vi "Autonomous Independent.vi"   [LabVIEW 2013]
doc: "This VI is called when autonomous begins, and will automatically be terminated when autonomous ends. You can carry out timed or sensor driven robot movement independently without needing to return to the caller."
uses:
  <vilib>/Rock Robotics/WPI/Relay/WPI_RelayValue.ctl
  <vilib>/Rock Robotics/WPI/Solenoid/WPI_SolenoidValue.ctl
  Robot Global Data.vi
  <vilib>/Rock Robotics/WPI/RobotDrive/WPI_RobotDriveGetSetRefNum.vi
  <vilib>/Rock Robotics/WPI/RobotDrive/WPI_RobotDriveArcadeDrive_Standard(NoSaturation).vi
  <vilib>/Rock Robotics/WPI/Solenoid/WPI_SolenoidSetEnum.vi
  <vilib>/Rock Robotics/WPI/Joystick/WPI_JoystickGetSetRefNum.vi
panel:
  # "Be sure to right-click and choose Data Operations>>Make Current Value default if you want to save the array values with the VI"
types:
  T1 = typedef "WPI_JoystickDevRef.ctl" = cluster{"Device":T2}
  T2 = typedef "WPI_JoystickDeviceEnum.ctl" = enum16{"USB 1", "USB 2", "USB 3", "USB 4", "Kinect 1", "Kinect 2"}
  T3 = cluster{"axis 1 (x)":dbl, "axis 2 (y)":dbl, "axis 3 (throttle)":dbl, "axis 4":dbl, "axis 5":dbl, "axis 6":dbl}
  T4 = typedef "WPI_RobotDriveDevRef.ctl" = cluster{"DevStatus":errorcluster, "Motors[]":T5[], "Square Inputs":bool, "Max Output":dbl, "Isochronous":bool}
  T5 = typedef "WPI_MotorControlDeviceRef.ctl" = cluster{"DeviceStatus":errorcluster, "Type":enum16{"PWM", "CAN"}, "PWM":cluster{"Digital Module":T6, "PWM Channel":T7, "DeadBand":T8}, "CAN":cluster{"Device Number":u8, "Control Mode":T9, "Semaphore":T10, "Max Vout":dbl}, "Invert":bool, "TransformRef":T11, "InvTransformRef":T11}
  T6 = typedef "FPGA_TypedefDigitalModule.ctl" = enum16{"Digital Module 1", "Digital Module 2"}
  T7 = typedef "FPGA_DIOPWMChannel.ctl" = enum8{"PWM 1", "PWM 2", "PWM 3", "PWM 4", "PWM 5", "PWM 6", "PWM 7", "PWM 8", "PWM 9", "PWM 10", "Invalid"}
  T8 = typedef "WPI_PWMDeadband.ctl" = cluster{"Name":string, "maxPositivePwm":i32, "minPositivePwm":i32, "centerPwm":i32, "maxNegativePwm":i32, "minNegativePwm":i32, "angularRange":u16}
  T9 = typedef "WPI_CANJaguar_ControlMode.ctl" = enum8{"Percent VBus", "Current", "Speed", "Position", "Voltage"}
  T10 = typedef "Semaphore RefNum" = refnum<k1>
  T11 = typedef "WPI_PWMTransform_ConPane.ctl" = refnum<vi>
  T12 = typedef "WPI_RelayDevRef.ctl" = cluster{"DevStatus":errorcluster, "Relay Channel":T13, "Digital Module":T6, "Relay Direction":T14}
  T13 = typedef "FPGA_DIORelayChannel.ctl" = enum8{"Relay 1", "Relay 2", "Relay 3", "Relay 4", "Relay 5", "Relay 6", "Relay 7", "Relay 8", "Invalid"}
  T14 = typedef "WPI_RelayDirection.ctl" = enum16{"Both directions", "Forward only", "Reverse only"}
  T15 = typedef "WPI_SolenoidDevRef.ctl" = cluster{"DevStatus":errorcluster, "Solenoid Module":T16, "Forward Solenoid Channel":T17, "Reverse Solenoid Channel":T17}
  T16 = typedef "FPGA_TypedefSolenoidModule.ctl" = enum16{"Solenoid Module 1", "Solenoid Module 2"}
  T17 = typedef "WPI_SolenoidChannel.ctl" = enum8{"Solenoid 1", "Solenoid 2", "Solenoid 3", "Solenoid 4", "Solenoid 5", "Solenoid 6", "Solenoid 7", "Solenoid 8", "Invalid"}
  T18 = typedef "WPI_SolenoidValue.ctl" = enum16{"Off", "On", "Forward", "Reverse"}
  T19 = typedef "WPI_RelayValue.ctl" = enum16{"Off", "On", "Forward", "Reverse"}
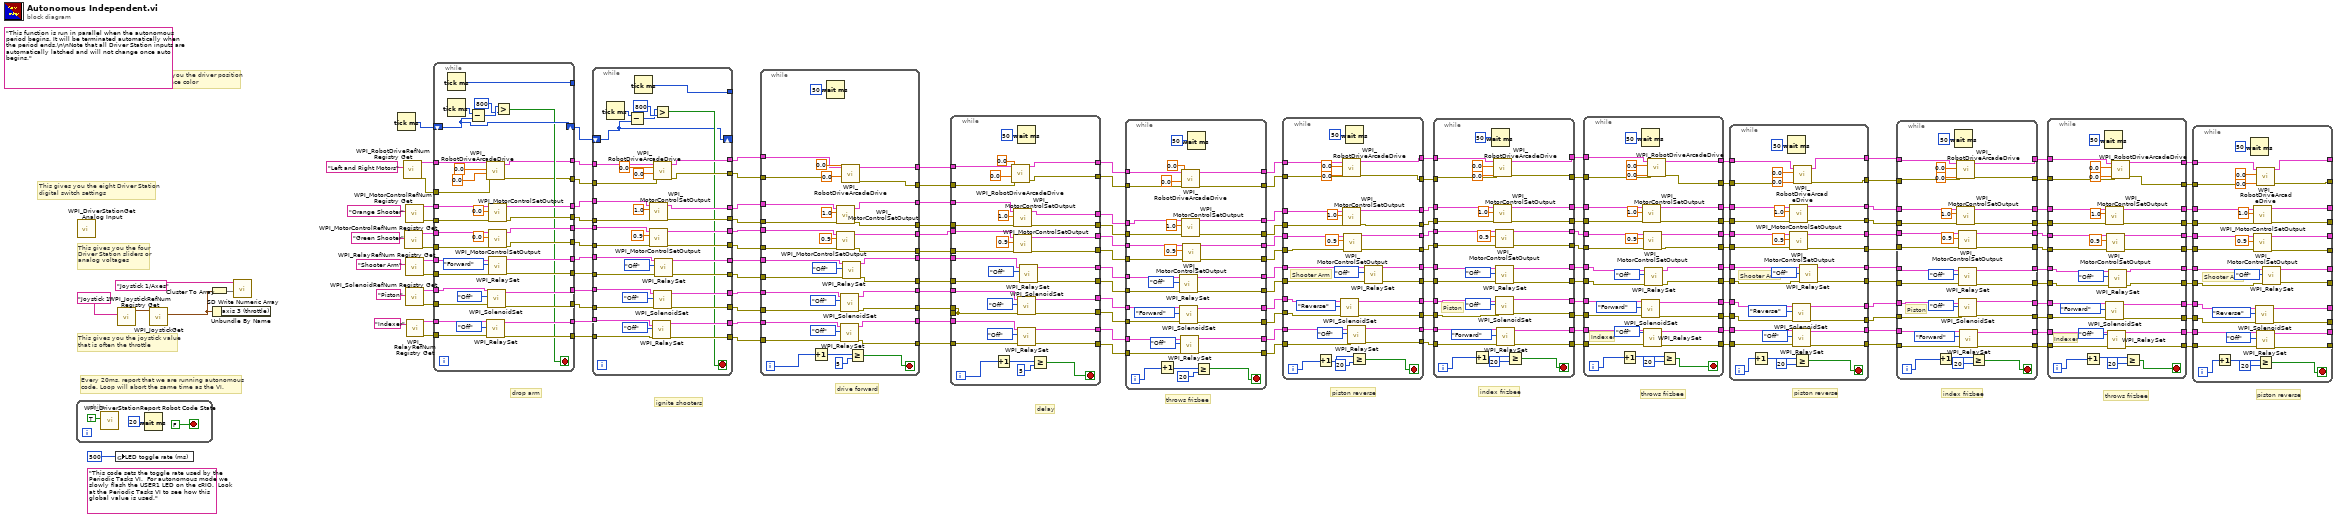
[diagram p0: block diagram]
diagram:
  (unwired) "This code sets the toggle rate used by the Periodic Tasks VI.  For autonomous mode we slowly flash the USER1 LED on the cRIO.  Look at the Periodic Tasks VI to see how this global value is used."
  (unwired) "This function is run in parallel when the autonomous period begins. It will be terminated automatically when the period ends.\n\nNote that all Driver Station inputs are automatically latched and will not change once auto begins."
  # "piston reverse"
  # "throws frizbee"
  # "index frizbee"
  # "drive forward"
  # "delay"
  # "ignite shooters"
  # "drop arm"
  # "piston reverse"
  # "throws frizbee"
  # "index frizbee"
  # "piston reverse"
  # "throws frizbee"
  # "This tells you the driver position\nand alliance color"
  # "Every 20ms, report that we are running autonomous\ncode. Loop will abort the same time as the VI."
  # "This gives you the joystick value\nthat is often the throttle"
  # "This gives you the eight Driver Station\ndigital switch settings"
  # "This gives you the four\nDriver Station sliders or\nanalog voltages"
  n1 = while {
    stop <- FALSE stop-if-true
    n2 = call <vilib>:"WPI_DriverStationReport Robot Code State.vi"("Autonomous"=TRUE) -> ()  [unwired: 10 in, 1 out]
    n3 = Wait (ms)(milliseconds to wait=u32 20) -> ()  [unwired: 1 out]
  }
  n4 = call <vilib>:"WPI_DriverStationGet Analog Input.vi"() -> ()  [unwired: 12 out]
  n5 = global write "Robot Global Data.vi" "LED toggle rate (ms)"(u32 500 ("LED ms toggle rate")) -> ()
  n6 = call <vilib>:"WPI_JoystickRefNum Registry Get.vi"("refnum name"="Joystick 1") -> ("JoystickDevRef"=w157:T1)  [unwired: 1 in, 9 out]
  n7 = call <vilib>:"WPI_JoystickGet.vi"("JoystickDevRef"=w157) -> ("Axes"=w154:T3)  [unwired: 1 in, 5 out]
  n8 = Cluster To Array(cluster=w154) -> (array=w155:dbl[])
  n9 = Unbundle By Name(w154) -> ()  [unwired: 1 out]
  n10 = call <vilib>:"SD Write Numeric Array.vi"("Numeric Array"=w155, "Name"="Joystick 1/Axes") -> ()  [unwired: 8 in, 2 out]
  n11 = Tick Count (ms)() -> (millisecond timer value=w148:u32)
  n12 = call <vilib>:"WPI_RobotDriveRefNum Registry Get.vi"("refnum name"="Left and Right Motors") -> ("error out"=w152:errorcluster, "RobotDriveDevRef"=w151:T4)  [unwired: 9 in]
  n13 = call <vilib>:"WPI_MotorControlRefNum Registry Get.vi"("refnum name"="Green Shooter") -> ("error out"=w138:errorcluster, "MotorControlDevRef"=w141:T5)  [unwired: 9 in]
  n14 = call <vilib>:"WPI_MotorControlRefNum Registry Get.vi"("refnum name"="Orange Shooter") -> ("error out"=w137:errorcluster, "MotorControlDevRef"=w140:T5)  [unwired: 9 in]
  n15 = call <vilib>:"WPI_RelayRefNum Registry Get.vi"("refnum name"="Shooter Arm") -> ("error out"=w139:errorcluster, "RelayDevRef"=w142:T12)  [unwired: 9 in]
  n16 = call <vilib>:"WPI_SolenoidRefNum Registry Get.vi"("refnum name"="Piston") -> ("error out"=w144:errorcluster, "SolenoidDevRef"=w143:T15)  [unwired: 9 in]
  n17 = call <vilib>:"WPI_RelayRefNum Registry Get.vi"("refnum name"="Indexer") -> ("error out"=w147:errorcluster, "RelayDevRef"=w146:T12)  [unwired: 9 in]
  n18 = while {
    tunnel: w137 -> [w198]
    tunnel: w138 -> [w197]
    tunnel: w139 -> [w196]
    tunnel: w140 -> [w188]
    tunnel: w141 -> [w185]
    tunnel: w142 -> [w195]
    tunnel: [w193] -> w129
    tunnel: [w192] -> w130
    tunnel: [w191] -> w128
    tunnel: [w190] -> w127
    tunnel: [w189] -> w126
    tunnel: w143 -> [w169]
    tunnel: w144 -> [w183]
    tunnel: [w182] -> w125
    tunnel: [w181] -> w124
    tunnel: w146 -> [w180]
    tunnel: [w178] -> w123
    tunnel: [w177] -> w122
    tunnel: w147 -> [w179]
    tunnel: [w187] -> w131
    shift-right: [w175] -> w61
    shift-left: w148 -> [w175]
    tunnel: [w171] -> _
    tunnel: w151 -> [w167]
    tunnel: [w166] -> w133
    tunnel: [w163] -> w132
    tunnel: w152 -> [w162]
    stop <- w172 stop-if-true
    n19 = Tick Count (ms)() -> (millisecond timer value=w170:u32)
    n20 = Tick Count (ms)() -> (millisecond timer value=w171:u32)
    n21 = Subtract(x=w170, y=w175) -> (x-y=w174:u32)
    n22 = call-poly <vilib>:"WPI_RobotDriveArcadeDrive.vi"("error in (no error)"=w162, "Y axis value"=0.0 ("X axis value"), "X axis value"=0.0, "RobotDriveDevRef"=w167) -> ("error out"=w163:errorcluster, "RobotDriveDevRef"=w166:T4)  [unwired: 5 in, 1 out]
    n23 = call <vilib>:"WPI_RelaySet.vi"("error in (no error)"=w179, "RelayValue"=WPI_RelayValue."Off", "RelayDevRef"=w180) -> ("error out"=w177:errorcluster, "RelayDevRef"=w178:T12)  [unwired: 7 in]
    n24 = call-poly <vilib>:"WPI_SolenoidSet.vi"("error in (no error)"=w183, "Value"=WPI_SolenoidValue."Off", "SolenoidDevRef"=w169) -> ("error out"=w181:errorcluster, "SolenoidDevRef"=w182:T15)  [unwired: 7 in]
    n25 = call <vilib>:"WPI_MotorControlSetOutput.vi"("error in (no error)"=w198, "Output"=0.0, "MotorControlDevRef"=w188) -> ("error out"=w192:errorcluster, "MotorControlDevRef"=w187:T5)  [unwired: 6 in, 1 out]
    n26 = call <vilib>:"WPI_MotorControlSetOutput.vi"("error in (no error)"=w197, "Output"=0.0, "MotorControlDevRef"=w185) -> ("error out"=w191:errorcluster, "MotorControlDevRef"=w193:T5)  [unwired: 6 in, 1 out]
    n27 = call <vilib>:"WPI_RelaySet.vi"("error in (no error)"=w196, "RelayValue"=WPI_RelayValue."Forward", "RelayDevRef"=w195) -> ("error out"=w189:errorcluster, "RelayDevRef"=w190:T12)  [unwired: 7 in]
    n28 = Greater?(x=w174, y=u32 800) -> (0:w172:bool)
  }
  n29 = while {
    tunnel: w131 -> [w233]
    tunnel: w130 -> [w232]
    tunnel: w129 -> [w231]
    tunnel: w128 -> [w230]
    tunnel: [w229] -> w42
    tunnel: [w228] -> w41
    tunnel: [w227] -> w39
    tunnel: [w226] -> w40
    tunnel: w127 -> [w222]
    tunnel: w126 -> [w221]
    tunnel: [w220] -> w51
    tunnel: [w219] -> w52
    tunnel: w125 -> [w218]
    tunnel: w124 -> [w217]
    tunnel: w123 -> [w216]
    tunnel: w122 -> [w215]
    tunnel: [w214] -> w60
    tunnel: [w213] -> w59
    tunnel: [w212] -> w56
    tunnel: [w211] -> w55
    tunnel: w133 -> [w210]
    tunnel: [w209] -> w44
    tunnel: w132 -> [w206]
    tunnel: [w205] -> w43
    tunnel: [w204] -> _
    shift-right: [w199] -> _
    shift-left: w61 -> [w199]
    stop <- w200 stop-if-true
    n30 = Tick Count (ms)() -> (millisecond timer value=w203:u32)
    n31 = Subtract(x=w203, y=w199) -> (x-y=w201:u32)
    n32 = Tick Count (ms)() -> (millisecond timer value=w204:u32)
    n33 = call <vilib>:"WPI_MotorControlSetOutput.vi"("error in (no error)"=w232, "Output"=1.0, "MotorControlDevRef"=w233) -> ("error out"=w228:errorcluster, "MotorControlDevRef"=w229:T5)  [unwired: 6 in, 1 out]
    n34 = call <vilib>:"WPI_MotorControlSetOutput.vi"("error in (no error)"=w230, "Output"=0.9, "MotorControlDevRef"=w231) -> ("error out"=w227:errorcluster, "MotorControlDevRef"=w226:T5)  [unwired: 6 in, 1 out]
    n35 = call <vilib>:"WPI_RelaySet.vi"("error in (no error)"=w215, "RelayValue"=WPI_RelayValue."Off", "RelayDevRef"=w216) -> ("error out"=w213:errorcluster, "RelayDevRef"=w214:T12)  [unwired: 7 in]
    n36 = call-poly <vilib>:"WPI_SolenoidSet.vi"("error in (no error)"=w217, "Value"=WPI_SolenoidValue."Off", "SolenoidDevRef"=w218) -> ("error out"=w212:errorcluster, "SolenoidDevRef"=w211:T15)  [unwired: 7 in]
    n37 = Greater?(x=w201, y=u32 800) -> (0:w200:bool)
    n38 = call-poly <vilib>:"WPI_RobotDriveArcadeDrive.vi"("error in (no error)"=w206, "Y axis value"=0.0, "X axis value"=0.0, "RobotDriveDevRef"=w210) -> ("error out"=w205:errorcluster, "RobotDriveDevRef"=w209:T4)  [unwired: 5 in, 1 out]
    n39 = call <vilib>:"WPI_RelaySet.vi"("error in (no error)"=w221, "RelayValue"=WPI_RelayValue."Off", "RelayDevRef"=w222) -> ("error out"=w219:errorcluster, "RelayDevRef"=w220:T12)  [unwired: 7 in]
  }
  n40 = while {
    tunnel: w60 -> [w264]
    tunnel: w59 -> [w263]
    tunnel: [w262] -> w58
    tunnel: [w261] -> w57
    tunnel: w56 -> [w260]
    tunnel: w55 -> [w259]
    tunnel: [w258] -> w54
    tunnel: [w257] -> w53
    tunnel: w52 -> [w256]
    tunnel: w51 -> [w255]
    tunnel: [w254] -> w50
    tunnel: [w253] -> w49
    tunnel: [w252] -> w48
    tunnel: [w251] -> w47
    tunnel: [w250] -> w46
    tunnel: [w249] -> w45
    tunnel: w44 -> [w247]
    tunnel: w43 -> [w246]
    tunnel: w42 -> [w245]
    tunnel: w41 -> [w244]
    tunnel: w40 -> [w243]
    tunnel: w39 -> [w242]
    tunnel: [w241] -> w38
    tunnel: [w240] -> w37
    i -> [w237]
    stop <- w236 stop-if-true
    n41 = Increment(x=w237) -> (x+1=w238:i32)
    n42 = Wait (ms)(milliseconds to wait=u32 50) -> ()  [unwired: 1 out]
    n43 = call <vilib>:"WPI_MotorControlSetOutput.vi"("error in (no error)"=w244, "Output"=1.0, "MotorControlDevRef"=w245) -> ("error out"=w249:errorcluster, "MotorControlDevRef"=w250:T5)  [unwired: 6 in, 1 out]
    n44 = call <vilib>:"WPI_MotorControlSetOutput.vi"("error in (no error)"=w242, "Output"=0.9, "MotorControlDevRef"=w243) -> ("error out"=w252:errorcluster, "MotorControlDevRef"=w251:T5)  [unwired: 6 in, 1 out]
    n45 = call <vilib>:"WPI_RelaySet.vi"("error in (no error)"=w263, "RelayValue"=WPI_RelayValue."Off", "RelayDevRef"=w264) -> ("error out"=w261:errorcluster, "RelayDevRef"=w262:T12)  [unwired: 7 in]
    n46 = call-poly <vilib>:"WPI_SolenoidSet.vi"("error in (no error)"=w260, "Value"=WPI_SolenoidValue."Off", "SolenoidDevRef"=w259) -> ("error out"=w257:errorcluster, "SolenoidDevRef"=w258:T15)  [unwired: 7 in]
    n47 = call-poly <vilib>:"WPI_RobotDriveArcadeDrive.vi"("error in (no error)"=w246, "Y axis value"=0.0, "X axis value"=0.0, "RobotDriveDevRef"=w247) -> ("error out"=w240:errorcluster, "RobotDriveDevRef"=w241:T4)  [unwired: 5 in, 1 out]
    n48 = call <vilib>:"WPI_RelaySet.vi"("error in (no error)"=w256, "RelayValue"=WPI_RelayValue."Off", "RelayDevRef"=w255) -> ("error out"=w253:errorcluster, "RelayDevRef"=w254:T12)  [unwired: 7 in]
    n49 = Greater Or Equal?(x=w238, y=5) -> (x >= y?=w236:bool)
  }
  n50 = while {
    tunnel: [w288] -> w102
    tunnel: [w289] -> w103
    tunnel: [w290] -> w104
    tunnel: [w291] -> w105
    tunnel: [w292] -> w106
    tunnel: [w293] -> w107
    tunnel: [w294] -> w108
    tunnel: [w295] -> w109
    tunnel: [w296] -> w110
    tunnel: [w297] -> w111
    tunnel: [w285] -> w112
    tunnel: [w284] -> w113
    tunnel: w38 -> [w283]
    tunnel: w37 -> [w282]
    tunnel: w45 -> [w281]
    tunnel: w46 -> [w280]
    tunnel: w48 -> [w279]
    tunnel: w47 -> [w278]
    tunnel: w49 -> [w277]
    tunnel: w50 -> [w276]
    tunnel: w54 -> [w275]
    tunnel: [w272] -> _
    tunnel: w58 -> [w274]
    tunnel: w57 -> [w273]
    tunnel: w53 -> [w272]
    i -> [w304]
    stop <- w303 stop-if-true
    n51 = Increment(x=w304) -> (x+1=w306:i32)
    n52 = call-poly <vilib>:"WPI_RobotDriveArcadeDrive.vi"("error in (no error)"=w282, "Y axis value"=0.0, "X axis value"=0.0, "RobotDriveDevRef"=w283) -> ("error out"=w284:errorcluster, "RobotDriveDevRef"=w285:T4)  [unwired: 5 in, 1 out]
    n53 = call <vilib>:"WPI_MotorControlSetOutput.vi"("error in (no error)"=w281, "Output"=1.0, "MotorControlDevRef"=w280) -> ("error out"=w289:errorcluster, "MotorControlDevRef"=w288:T5)  [unwired: 6 in, 1 out]
    n54 = call <vilib>:"WPI_MotorControlSetOutput.vi"("error in (no error)"=w279, "Output"=0.9, "MotorControlDevRef"=w278) -> ("error out"=w291:errorcluster, "MotorControlDevRef"=w290:T5)  [unwired: 6 in, 1 out]
    n55 = Wait (ms)(milliseconds to wait=u32 50) -> ()  [unwired: 1 out]
    n56 = call <vilib>:"WPI_RelaySet.vi"("error in (no error)"=w273, "RelayValue"=WPI_RelayValue."Off", "RelayDevRef"=w274) -> ("error out"=w297:errorcluster, "RelayDevRef"=w296:T12)  [unwired: 7 in]
    n57 = call-poly <vilib>:"WPI_SolenoidSet.vi"("error in (no error)"=w272, "Value"=WPI_SolenoidValue."Off", "SolenoidDevRef"=w275) -> ("error out"=w295:errorcluster, "SolenoidDevRef"=w294:T15)  [unwired: 7 in]
    n58 = call <vilib>:"WPI_RelaySet.vi"("error in (no error)"=w277, "RelayValue"=WPI_RelayValue."Off", "RelayDevRef"=w276) -> ("error out"=w293:errorcluster, "RelayDevRef"=w292:T12)  [unwired: 7 in]
    n59 = Greater Or Equal?(x=w306, y=5) -> (x >= y?=w303:bool)
  }
  n60 = while {
    tunnel: w104 -> [w328]
    tunnel: w103 -> [w343]
    tunnel: w105 -> [w342]
    tunnel: w106 -> [w326]
    tunnel: [w324] -> w62
    tunnel: w107 -> [w325]
    tunnel: [w323] -> w70
    tunnel: [w341] -> w68
    tunnel: [w340] -> w69
    tunnel: [w339] -> w66
    tunnel: [w338] -> w67
    tunnel: w108 -> [w315]
    tunnel: w109 -> [w337]
    tunnel: [w336] -> w64
    tunnel: [w335] -> w65
    tunnel: [w319] -> w78
    tunnel: w110 -> [w321]
    tunnel: w111 -> [w320]
    tunnel: [w318] -> w79
    tunnel: w102 -> [w330]
    tunnel: w112 -> [w313]
    tunnel: w113 -> [w312]
    tunnel: [w311] -> w114
    tunnel: [w310] -> w115
    i -> [w334]
    stop <- w331 stop-if-true
    n61 = Increment(x=w334) -> (x+1=w333:i32)
    n62 = call <vilib>:"WPI_RelaySet.vi"("error in (no error)"=w325, "RelayValue"=WPI_RelayValue."Off", "RelayDevRef"=w326) -> ("error out"=w323:errorcluster, "RelayDevRef"=w324:T12)  [unwired: 7 in]
    n63 = call-poly <vilib>:"WPI_SolenoidSet.vi"("error in (no error)"=w337, "Value"=WPI_SolenoidValue."Forward", "SolenoidDevRef"=w315) -> ("error out"=w335:errorcluster, "SolenoidDevRef"=w336:T15)  [unwired: 7 in]
    n64 = call <vilib>:"WPI_RelaySet.vi"("error in (no error)"=w320, "RelayValue"=WPI_RelayValue."Off", "RelayDevRef"=w321) -> ("error out"=w318:errorcluster, "RelayDevRef"=w319:T12)  [unwired: 7 in]
    n65 = call-poly <vilib>:"WPI_RobotDriveArcadeDrive.vi"("error in (no error)"=w312, "Y axis value"=0.0, "X axis value"=0.0, "RobotDriveDevRef"=w313) -> ("error out"=w310:errorcluster, "RobotDriveDevRef"=w311:T4)  [unwired: 5 in, 1 out]
    n66 = call <vilib>:"WPI_MotorControlSetOutput.vi"("error in (no error)"=w343, "Output"=1.0, "MotorControlDevRef"=w330) -> ("error out"=w338:errorcluster, "MotorControlDevRef"=w339:T5)  [unwired: 6 in, 1 out]
    n67 = call <vilib>:"WPI_MotorControlSetOutput.vi"("error in (no error)"=w342, "Output"=0.9, "MotorControlDevRef"=w328) -> ("error out"=w340:errorcluster, "MotorControlDevRef"=w341:T5)  [unwired: 6 in, 1 out]
    n68 = Wait (ms)(milliseconds to wait=u32 50) -> ()  [unwired: 1 out]
    n69 = Greater Or Equal?(x=w333, y=20) -> (x >= y?=w331:bool)
  }
  n70 = while {
    tunnel: w62 -> [w357]
    tunnel: [w355] -> w63
    tunnel: w64 -> [w352]
    tunnel: w65 -> [w376]
    tunnel: w66 -> [w366]
    tunnel: w67 -> [w365]
    tunnel: w68 -> [w364]
    tunnel: w69 -> [w378]
    tunnel: w70 -> [w356]
    tunnel: [w354] -> w75
    tunnel: [w377] -> w76
    tunnel: [w375] -> w77
    tunnel: [w374] -> w71
    tunnel: [w373] -> w74
    tunnel: [w372] -> w72
    tunnel: [w371] -> w73
    tunnel: [w359] -> w80
    tunnel: w78 -> [w361]
    tunnel: [w358] -> w81
    tunnel: w79 -> [w360]
    tunnel: w114 -> [w350]
    tunnel: w115 -> [w349]
    tunnel: [w346] -> w116
    tunnel: [w345] -> w117
    i -> [w370]
    stop <- w368 stop-if-true
    # "Shooter Arm"
    n71 = Increment(x=w370) -> (x+1=w369:i32)
    n72 = call-poly <vilib>:"WPI_SolenoidSet.vi"("error in (no error)"=w376, "Value"=WPI_SolenoidValue."Reverse", "SolenoidDevRef"=w352) -> ("error out"=w375:errorcluster, "SolenoidDevRef"=w377:T15)  [unwired: 7 in]
    n73 = call-poly <vilib>:"WPI_RobotDriveArcadeDrive.vi"("error in (no error)"=w349, "Y axis value"=0.0, "X axis value"=0.0, "RobotDriveDevRef"=w350) -> ("error out"=w345:errorcluster, "RobotDriveDevRef"=w346:T4)  [unwired: 5 in, 1 out]
    n74 = call <vilib>:"WPI_MotorControlSetOutput.vi"("error in (no error)"=w365, "Output"=1.0, "MotorControlDevRef"=w366) -> ("error out"=w373:errorcluster, "MotorControlDevRef"=w374:T5)  [unwired: 6 in, 1 out]
    n75 = call <vilib>:"WPI_MotorControlSetOutput.vi"("error in (no error)"=w378, "Output"=0.9, "MotorControlDevRef"=w364) -> ("error out"=w371:errorcluster, "MotorControlDevRef"=w372:T5)  [unwired: 6 in, 1 out]
    n76 = Wait (ms)(milliseconds to wait=u32 50) -> ()  [unwired: 1 out]
    n77 = call <vilib>:"WPI_RelaySet.vi"("error in (no error)"=w360, "RelayValue"=WPI_RelayValue."Off", "RelayDevRef"=w361) -> ("error out"=w358:errorcluster, "RelayDevRef"=w359:T12)  [unwired: 7 in]
    n78 = Greater Or Equal?(x=w369, y=20) -> (x >= y?=w368:bool)
    n79 = call <vilib>:"WPI_RelaySet.vi"("error in (no error)"=w356, "RelayValue"=WPI_RelayValue."Off", "RelayDevRef"=w357) -> ("error out"=w354:errorcluster, "RelayDevRef"=w355:T12)  [unwired: 7 in]
  }
  n80 = while {
    tunnel: w63 -> [w392]
    tunnel: [w389] -> w90
    tunnel: w71 -> [w398]
    tunnel: w72 -> [w400]
    tunnel: w73 -> [w415]
    tunnel: w74 -> [w399]
    tunnel: w75 -> [w391]
    tunnel: [w390] -> w91
    tunnel: w76 -> [w387]
    tunnel: w77 -> [w395]
    tunnel: [w394] -> w84
    tunnel: [w393] -> w85
    tunnel: [w414] -> w95
    tunnel: [w413] -> w94
    tunnel: [w412] -> w93
    tunnel: [w411] -> w92
    tunnel: w80 -> [w410]
    tunnel: w81 -> [w409]
    tunnel: [w408] -> w82
    tunnel: [w407] -> w83
    tunnel: w116 -> [w383]
    tunnel: w117 -> [w382]
    tunnel: [w381] -> w118
    tunnel: [w380] -> w119
    i -> [w404]
    stop <- w401 stop-if-true
    # "Piston"
    n81 = Increment(x=w404) -> (x+1=w403:i32)
    n82 = Wait (ms)(milliseconds to wait=u32 50) -> ()  [unwired: 1 out]
    n83 = call-poly <vilib>:"WPI_RobotDriveArcadeDrive.vi"("error in (no error)"=w382, "Y axis value"=0.0, "X axis value"=0.0, "RobotDriveDevRef"=w383) -> ("error out"=w380:errorcluster, "RobotDriveDevRef"=w381:T4)  [unwired: 5 in, 1 out]
    n84 = call <vilib>:"WPI_MotorControlSetOutput.vi"("error in (no error)"=w399, "Output"=1.0, "MotorControlDevRef"=w398) -> ("error out"=w413:errorcluster, "MotorControlDevRef"=w414:T5)  [unwired: 6 in, 1 out]
    n85 = call <vilib>:"WPI_MotorControlSetOutput.vi"("error in (no error)"=w415, "Output"=0.9, "MotorControlDevRef"=w400) -> ("error out"=w411:errorcluster, "MotorControlDevRef"=w412:T5)  [unwired: 6 in, 1 out]
    n86 = call <vilib>:"WPI_RelaySet.vi"("error in (no error)"=w391, "RelayValue"=WPI_RelayValue."Off", "RelayDevRef"=w392) -> ("error out"=w390:errorcluster, "RelayDevRef"=w389:T12)  [unwired: 7 in]
    n87 = call-poly <vilib>:"WPI_SolenoidSet.vi"("error in (no error)"=w395, "Value"=WPI_SolenoidValue."Off", "SolenoidDevRef"=w387) -> ("error out"=w393:errorcluster, "SolenoidDevRef"=w394:T15)  [unwired: 7 in]
    n88 = call <vilib>:"WPI_RelaySet.vi"("error in (no error)"=w409, "RelayValue"=WPI_RelayValue."Forward", "RelayDevRef"=w410) -> ("error out"=w407:errorcluster, "RelayDevRef"=w408:T12)  [unwired: 7 in]
    n89 = Greater Or Equal?(x=w403, y=20) -> (x >= y?=w401:bool)
  }
  n90 = while {
    tunnel: [w426] -> w88
    tunnel: w82 -> [w428]
    tunnel: [w425] -> w89
    tunnel: w83 -> [w427]
    tunnel: w84 -> [w423]
    tunnel: w85 -> [w451]
    tunnel: [w450] -> w86
    tunnel: [w449] -> w87
    tunnel: w90 -> [w433]
    tunnel: [w432] -> w100
    tunnel: w91 -> [w431]
    tunnel: [w430] -> w101
    tunnel: w92 -> [w448]
    tunnel: w93 -> [w436]
    tunnel: w94 -> [w437]
    tunnel: w95 -> [w438]
    tunnel: [w446] -> w98
    tunnel: [w445] -> w99
    tunnel: [w444] -> w97
    tunnel: [w443] -> w96
    tunnel: w118 -> [w419]
    tunnel: w119 -> [w418]
    tunnel: [w417] -> w120
    tunnel: [w416] -> w121
    i -> [w442]
    stop <- w439 stop-if-true
    # "Indexer"
    n91 = Increment(x=w442) -> (x+1=w441:i32)
    n92 = Wait (ms)(milliseconds to wait=u32 50) -> ()  [unwired: 1 out]
    n93 = call-poly <vilib>:"WPI_SolenoidSet.vi"("error in (no error)"=w451, "Value"=WPI_SolenoidValue."Forward", "SolenoidDevRef"=w423) -> ("error out"=w449:errorcluster, "SolenoidDevRef"=w450:T15)  [unwired: 7 in]
    n94 = call <vilib>:"WPI_MotorControlSetOutput.vi"("error in (no error)"=w437, "Output"=1.0, "MotorControlDevRef"=w438) -> ("error out"=w444:errorcluster, "MotorControlDevRef"=w443:T5)  [unwired: 6 in, 1 out]
    n95 = call <vilib>:"WPI_MotorControlSetOutput.vi"("error in (no error)"=w448, "Output"=0.9, "MotorControlDevRef"=w436) -> ("error out"=w446:errorcluster, "MotorControlDevRef"=w445:T5)  [unwired: 6 in, 1 out]
    n96 = call <vilib>:"WPI_RelaySet.vi"("error in (no error)"=w427, "RelayValue"=WPI_RelayValue."Off", "RelayDevRef"=w428) -> ("error out"=w425:errorcluster, "RelayDevRef"=w426:T12)  [unwired: 7 in]
    n97 = call <vilib>:"WPI_RelaySet.vi"("error in (no error)"=w431, "RelayValue"=WPI_RelayValue."Off", "RelayDevRef"=w433) -> ("error out"=w430:errorcluster, "RelayDevRef"=w432:T12)  [unwired: 7 in]
    n98 = call-poly <vilib>:"WPI_RobotDriveArcadeDrive.vi"("error in (no error)"=w418, "Y axis value"=0.0, "X axis value"=0.0, "RobotDriveDevRef"=w419) -> ("error out"=w416:errorcluster, "RobotDriveDevRef"=w417:T4)  [unwired: 5 in, 1 out]
    n99 = Greater Or Equal?(x=w441, y=20) -> (x >= y?=w439:bool)
  }
  n100 = while {
    tunnel: w86 -> [w459]
    tunnel: w87 -> [w487]
    tunnel: w88 -> [w464]
    tunnel: w89 -> [w462]
    tunnel: [w486] -> w4
    tunnel: [w485] -> w3
    tunnel: w96 -> [w473]
    tunnel: w97 -> [w472]
    tunnel: w98 -> [w484]
    tunnel: w99 -> [w474]
    tunnel: [w483] -> w8
    tunnel: [w482] -> w7
    tunnel: [w481] -> w9
    tunnel: [w480] -> w10
    tunnel: [w467] -> w6
    tunnel: w100 -> [w469]
    tunnel: [w466] -> w5
    tunnel: w101 -> [w468]
    tunnel: [w463] -> w2
    tunnel: [w461] -> w1
    tunnel: w120 -> [w455]
    tunnel: w121 -> [w454]
    tunnel: [w453] -> w12
    tunnel: [w452] -> w11
    i -> [w478]
    stop <- w475 stop-if-true
    # "Shooter Arm"
    n101 = Increment(x=w478) -> (x+1=w477:i32)
    n102 = Wait (ms)(milliseconds to wait=u32 50) -> ()  [unwired: 1 out]
    n103 = call <vilib>:"WPI_MotorControlSetOutput.vi"("error in (no error)"=w472, "Output"=1.0, "MotorControlDevRef"=w473) -> ("error out"=w481:errorcluster, "MotorControlDevRef"=w480:T5)  [unwired: 6 in, 1 out]
    n104 = call <vilib>:"WPI_MotorControlSetOutput.vi"("error in (no error)"=w484, "Output"=0.9, "MotorControlDevRef"=w474) -> ("error out"=w482:errorcluster, "MotorControlDevRef"=w483:T5)  [unwired: 6 in, 1 out]
    n105 = call-poly <vilib>:"WPI_SolenoidSet.vi"("error in (no error)"=w487, "Value"=WPI_SolenoidValue."Reverse", "SolenoidDevRef"=w459) -> ("error out"=w485:errorcluster, "SolenoidDevRef"=w486:T15)  [unwired: 7 in]
    n106 = call <vilib>:"WPI_RelaySet.vi"("error in (no error)"=w462, "RelayValue"=WPI_RelayValue."Off", "RelayDevRef"=w464) -> ("error out"=w461:errorcluster, "RelayDevRef"=w463:T12)  [unwired: 7 in]
    n107 = call-poly <vilib>:"WPI_RobotDriveArcadeDrive.vi"("error in (no error)"=w454, "Y axis value"=0.0, "X axis value"=0.0, "RobotDriveDevRef"=w455) -> ("error out"=w452:errorcluster, "RobotDriveDevRef"=w453:T4)  [unwired: 5 in, 1 out]
    n108 = Greater Or Equal?(x=w477, y=20) -> (x >= y?=w475:bool)
    n109 = call <vilib>:"WPI_RelaySet.vi"("error in (no error)"=w468, "RelayValue"=WPI_RelayValue."Off", "RelayDevRef"=w469) -> ("error out"=w466:errorcluster, "RelayDevRef"=w467:T12)  [unwired: 7 in]
  }
  n110 = while {
    tunnel: w6 -> [w500]
    tunnel: [w497] -> w28
    tunnel: w10 -> [w506]
    tunnel: w8 -> [w508]
    tunnel: w7 -> [w523]
    tunnel: w9 -> [w507]
    tunnel: w5 -> [w499]
    tunnel: [w498] -> w27
    tunnel: w4 -> [w495]
    tunnel: w3 -> [w503]
    tunnel: [w502] -> w34
    tunnel: [w501] -> w33
    tunnel: [w522] -> w23
    tunnel: [w521] -> w24
    tunnel: [w520] -> w25
    tunnel: [w519] -> w26
    tunnel: w2 -> [w518]
    tunnel: w1 -> [w517]
    tunnel: [w516] -> w36
    tunnel: [w515] -> w35
    tunnel: w12 -> [w491]
    tunnel: w11 -> [w490]
    tunnel: [w489] -> w16
    tunnel: [w488] -> w15
    i -> [w512]
    stop <- w509 stop-if-true
    # "Piston"
    n111 = Increment(x=w512) -> (x+1=w511:i32)
    n112 = Wait (ms)(milliseconds to wait=u32 50) -> ()  [unwired: 1 out]
    n113 = call-poly <vilib>:"WPI_RobotDriveArcadeDrive.vi"("error in (no error)"=w490, "Y axis value"=0.0, "X axis value"=0.0, "RobotDriveDevRef"=w491) -> ("error out"=w488:errorcluster, "RobotDriveDevRef"=w489:T4)  [unwired: 5 in, 1 out]
    n114 = call <vilib>:"WPI_MotorControlSetOutput.vi"("error in (no error)"=w507, "Output"=1.0, "MotorControlDevRef"=w506) -> ("error out"=w521:errorcluster, "MotorControlDevRef"=w522:T5)  [unwired: 6 in, 1 out]
    n115 = call <vilib>:"WPI_MotorControlSetOutput.vi"("error in (no error)"=w523, "Output"=0.9, "MotorControlDevRef"=w508) -> ("error out"=w519:errorcluster, "MotorControlDevRef"=w520:T5)  [unwired: 6 in, 1 out]
    n116 = call <vilib>:"WPI_RelaySet.vi"("error in (no error)"=w499, "RelayValue"=WPI_RelayValue."Off", "RelayDevRef"=w500) -> ("error out"=w498:errorcluster, "RelayDevRef"=w497:T12)  [unwired: 7 in]
    n117 = call-poly <vilib>:"WPI_SolenoidSet.vi"("error in (no error)"=w503, "Value"=WPI_SolenoidValue."Off", "SolenoidDevRef"=w495) -> ("error out"=w501:errorcluster, "SolenoidDevRef"=w502:T15)  [unwired: 7 in]
    n118 = call <vilib>:"WPI_RelaySet.vi"("error in (no error)"=w517, "RelayValue"=WPI_RelayValue."Forward", "RelayDevRef"=w518) -> ("error out"=w515:errorcluster, "RelayDevRef"=w516:T12)  [unwired: 7 in]
    n119 = Greater Or Equal?(x=w511, y=20) -> (x >= y?=w509:bool)
  }
  n120 = while {
    tunnel: [w534] -> w30
    tunnel: w36 -> [w536]
    tunnel: [w533] -> w29
    tunnel: w35 -> [w535]
    tunnel: w34 -> [w531]
    tunnel: w33 -> [w559]
    tunnel: [w558] -> w32
    tunnel: [w557] -> w31
    tunnel: w28 -> [w541]
    tunnel: [w540] -> w18
    tunnel: w27 -> [w539]
    tunnel: [w538] -> w17
    tunnel: w26 -> [w556]
    tunnel: w25 -> [w544]
    tunnel: w24 -> [w545]
    tunnel: w23 -> [w546]
    tunnel: [w554] -> w20
    tunnel: [w553] -> w19
    tunnel: [w552] -> w21
    tunnel: [w551] -> w22
    tunnel: w16 -> [w527]
    tunnel: w15 -> [w526]
    tunnel: [w525] -> w14
    tunnel: [w524] -> w13
    i -> [w550]
    stop <- w547 stop-if-true
    # "Indexer"
    n121 = Increment(x=w550) -> (x+1=w549:i32)
    n122 = Wait (ms)(milliseconds to wait=u32 50) -> ()  [unwired: 1 out]
    n123 = call-poly <vilib>:"WPI_SolenoidSet.vi"("error in (no error)"=w559, "Value"=WPI_SolenoidValue."Forward", "SolenoidDevRef"=w531) -> ("error out"=w557:errorcluster, "SolenoidDevRef"=w558:T15)  [unwired: 7 in]
    n124 = call <vilib>:"WPI_MotorControlSetOutput.vi"("error in (no error)"=w545, "Output"=1.0, "MotorControlDevRef"=w546) -> ("error out"=w552:errorcluster, "MotorControlDevRef"=w551:T5)  [unwired: 6 in, 1 out]
    n125 = call <vilib>:"WPI_MotorControlSetOutput.vi"("error in (no error)"=w556, "Output"=0.9, "MotorControlDevRef"=w544) -> ("error out"=w554:errorcluster, "MotorControlDevRef"=w553:T5)  [unwired: 6 in, 1 out]
    n126 = call <vilib>:"WPI_RelaySet.vi"("error in (no error)"=w535, "RelayValue"=WPI_RelayValue."Off", "RelayDevRef"=w536) -> ("error out"=w533:errorcluster, "RelayDevRef"=w534:T12)  [unwired: 7 in]
    n127 = call <vilib>:"WPI_RelaySet.vi"("error in (no error)"=w539, "RelayValue"=WPI_RelayValue."Off", "RelayDevRef"=w541) -> ("error out"=w538:errorcluster, "RelayDevRef"=w540:T12)  [unwired: 7 in]
    n128 = call-poly <vilib>:"WPI_RobotDriveArcadeDrive.vi"("error in (no error)"=w526, "Y axis value"=0.0, "X axis value"=0.0, "RobotDriveDevRef"=w527) -> ("error out"=w524:errorcluster, "RobotDriveDevRef"=w525:T4)  [unwired: 5 in, 1 out]
    n129 = Greater Or Equal?(x=w549, y=20) -> (x >= y?=w547:bool)
  }
  n130 = while {
    tunnel: w32 -> [w567]
    tunnel: w31 -> [w595]
    tunnel: w30 -> [w572]
    tunnel: w29 -> [w570]
    tunnel: [w594] -> _
    tunnel: [w593] -> _
    tunnel: w22 -> [w581]
    tunnel: w21 -> [w580]
    tunnel: w20 -> [w592]
    tunnel: w19 -> [w582]
    tunnel: [w591] -> _
    tunnel: [w590] -> _
    tunnel: [w589] -> _
    tunnel: [w588] -> _
    tunnel: [w575] -> _
    tunnel: w18 -> [w577]
    tunnel: [w574] -> _
    tunnel: w17 -> [w576]
    tunnel: [w571] -> _
    tunnel: [w569] -> _
    tunnel: w14 -> [w563]
    tunnel: w13 -> [w562]
    tunnel: [w561] -> _
    tunnel: [w560] -> _
    i -> [w586]
    stop <- w583 stop-if-true
    # "Shooter Arm"
    n131 = Increment(x=w586) -> (x+1=w585:i32)
    n132 = Wait (ms)(milliseconds to wait=u32 50) -> ()  [unwired: 1 out]
    n133 = call <vilib>:"WPI_MotorControlSetOutput.vi"("error in (no error)"=w580, "Output"=1.0, "MotorControlDevRef"=w581) -> ("error out"=w589:errorcluster, "MotorControlDevRef"=w588:T5)  [unwired: 6 in, 1 out]
    n134 = call <vilib>:"WPI_MotorControlSetOutput.vi"("error in (no error)"=w592, "Output"=0.9, "MotorControlDevRef"=w582) -> ("error out"=w590:errorcluster, "MotorControlDevRef"=w591:T5)  [unwired: 6 in, 1 out]
    n135 = call-poly <vilib>:"WPI_SolenoidSet.vi"("error in (no error)"=w595, "Value"=WPI_SolenoidValue."Reverse", "SolenoidDevRef"=w567) -> ("error out"=w593:errorcluster, "SolenoidDevRef"=w594:T15)  [unwired: 7 in]
    n136 = call <vilib>:"WPI_RelaySet.vi"("error in (no error)"=w570, "RelayValue"=WPI_RelayValue."Off", "RelayDevRef"=w572) -> ("error out"=w569:errorcluster, "RelayDevRef"=w571:T12)  [unwired: 7 in]
    n137 = call-poly <vilib>:"WPI_RobotDriveArcadeDrive.vi"("error in (no error)"=w562, "Y axis value"=0.0, "X axis value"=0.0, "RobotDriveDevRef"=w563) -> ("error out"=w560:errorcluster, "RobotDriveDevRef"=w561:T4)  [unwired: 5 in, 1 out]
    n138 = Greater Or Equal?(x=w585, y=20) -> (x >= y?=w583:bool)
    n139 = call <vilib>:"WPI_RelaySet.vi"("error in (no error)"=w576, "RelayValue"=WPI_RelayValue."Off", "RelayDevRef"=w577) -> ("error out"=w574:errorcluster, "RelayDevRef"=w575:T12)  [unwired: 7 in]
  }
